vi "FPGA Top - Packet RX Only.vi"() -> ()   [LabVIEW 2017, in "My Network FPGA v1.lvlib"]
uses:
  My Network FPGA v1.lvlib
  <instrlib>/_niInstr/Network/Types/v1/IPv4 Address.ctl
  <instrlib>/_niInstr/Network/Types/v1/MAC Address.ctl
  <instrlib>/_niInstr/Network/Ethernet/MAC/CLIP/v1/Resources.ctl
  <vilib>/Platform/TimedLoop/XDataNode/timing_clust.ctl
  <vilib>/Platform/TimedLoop/XDataNode/nitl_modes.ctl
  <vilib>/Platform/TimedLoop/XDataNode/wakeup.ctl
  <vilib>/rvi/Emulation/niFpgaSctlEmulationGetInTimedLoop.vi
  <vilib>/rvi/Emulation/niFpgaEmulationReportErrorSimple.vi
  <vilib>/rvi/Emulation/niFpgaGetClockAttributes.vi
  <vilib>/rvi/Emulation/niFpgaCriticalErrorInLSC.vi
  <instrlib>/_niInstr/Network/IPv4/UDP/Data Stream/v1/Read Data Stream.vi
  <vilib>/rvi/DataTransferAndStorage/Container/Common/niFpgaContainerExecOnDevCompGetState.vi
  <vilib>/rvi/errors/niFpgaSetErrorForExecOnDevCompSimple.vi
  <vilib>/rvi/eio/common/nirviEmuReportErrorAndStop.vi
  <vilib>/rvi/interface/RandomDataEmulation/nirviRandomDataAcquireLock.vi
  <vilib>/rvi/interface/RandomDataEmulation/nirviRandomDataQueueStore.vi
  <vilib>/rvi/interface/RandomDataEmulation/nirviRandomDataReleaseLock.vi
  <vilib>/rvi/interface/RandomDataEmulation/nirviFPGAContextMergeError.vi
  <vilib>/rvi/interface/RandomDataEmulation/nirviRandomDataCheckExitLoopConditions.vi
  <vilib>/express/rvi/timingcommon/nirviCommon.vi
  <vilib>/rvi/interface/RandomDataEmulation/niFpgaRandomDataHandleErrors.vi
  <vilib>/rvi/eio/common/nirviEmuTemplateMethod_errors.vi
  <vilib>/platform/TimedLoop/XDataNode/XDataNode.xnode
  <vilib>/rvi/DataTransferAndStorage/Container/XNode/niFpgaContainer.xnode
  <vilib>/rvi/FIFO/Fifo_Resource/niFpgaFifoEmulationRefInMultiElement.vi
  <vilib>/eio/EIONode/EIONode.xnode
  <instrlib>/_niInstr/Network/Ethernet/MAC/CLIP/v1/niInstr Ethernet MAC - CLIP v1.lvclass
  <vilib>/Platform/TimedLoop/XDataNode/XDNodeRunTimeDep.lvlib
  <instrlib>/_niInstr/Network/IPv4/UDP/FPGA/v1/niInstr IPv4 UDP FPGA v1.lvlib
  <instrlib>/_niInstr/Network/IPv4/FPGA/v1/niInstr IPv4 FPGA v1.lvlib
  <instrlib>/_niInstr/Network/Ethernet/Utility/v1/FPGA/niInstr Ethernet Utilities FPGA v1.lvlib
  <instrlib>/_niInstr/Network/IPv4/UDP/Data Stream/v1/niInstr IPv4 UDP Data Stream v1.lvclass
  <instrlib>/_niInstr/Network/Ethernet/ARP/v1/FPGA/niInstr Network ARP FPGA v1.lvlib
  <instrlib>/_niInstr/Network/Types/v1/niInstr Network Types v1.lvlib
panel:
  out "aBlockLockPort0":bool
  out "aBlockLockPort1":bool
  out "mgtrefclks_locked":bool
  out "mgtrefclks_valid":bool
  out "posc_complete":bool
  out "sPort0_Power_Good":bool
  out "sPort1_Power_Good":bool
  out "signal_detect_Port0":bool
  out "signal_detect_Port1":bool
  in  "disable IP filtering":bool
  out "byte enables":bool[](array[boolean])
  out "data":u8[](array[numeric])
  in  "Promiscuous?":bool
  in  "MAC local address":T1=[0, 128, 47, 0, 0, 1] format="%.0x"
  in  "IPv4 local address":T2=[0, 0, 0, 0]
  in  "UDP destination port":u16=35311
  # "Network Configuration"
  # "Received Data"
  # "Status"
  # "00802F000001x2^0"
  # "Also see Port 0 RX FIFO"
  # "License Note\nThis example makes use of code under the LGPLv2 license in the Socketed CLIP to support 10 Gigabit Ethernet.  You may find the source and build instructions for this component in the CLIP directory."
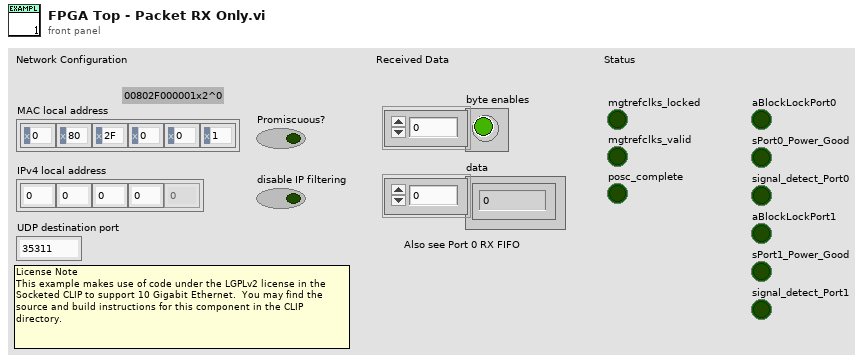
[diagram p1: front panel]
types:
  T1 = typedef "niInstr Network Types v1.lvlib/MAC Address.ctl" = u8[]
  T2 = typedef "niInstr Network Types v1.lvlib/IPv4 Address.ctl" = u8[]
  T3 = typedef "niInstr Ethernet MAC - CLIP v1.lvclass/Resources.ctl" = cluster{"RX":cluster{"TData":refnum<k21>, "TValid":refnum<k21>, "TKeep":refnum<k21>, "TLast":refnum<k21>, "TUser":refnum<k21>}, "TX":cluster{"TData":refnum<k21>, "TValid":refnum<k21>, "TKeep":refnum<k21>, "TLast":refnum<k21>, "TReady":refnum<k21>}, "Pause resources":cluster{"cPauseValuePort":refnum<k21>, "cPauseReqPort":refnum<k21>}, "MAC Clock":refnum<k21>}
  T4 = typedef "XDNodeRunTimeDep.lvlib/timing_clust.ctl" = cluster{"Expected End [f-1]":u64, "Actual End [f-1]":u64, "Finished Late? [f-1]":bool, "Expected End [i-1]":u64, "Actual End [i-1]":u64, "Finished Late? [i-1]":bool, "Expected Start [i]":u64, "Actual Start [i]":u64, "Expected Start [f]":u64, "Actual Start [f]":u64, "Source Name":string, "Structure Name":string, "Period":i64, "Deadline":i64, "Offset":i64, "Start":i64, "Priority":i32, "Timeout":i32, "Mode":T5, "Wakeup Reason":T6, "Error":errorcluster, "Source Type":string, "Secondary Source Type":string, "Global End Time":u64, "Global Start Time":u64, "Frame Duration":u64, "Iteration Duration":u64, "Assigned CPU":i32, "I/O Scan Engine Mode":u32}
  T5 = typedef "XDNodeRunTimeDep.lvlib/nitl_modes.ctl" = enum32{"No Change", "Process missed periods, maintain original phase", "Discard missed periods, maintain original phase", "Process missed periods, ignore original phase", "Discard missed periods, ignore original phase"}
  T6 = typedef "XDNodeRunTimeDep.lvlib/wakeup.ctl" = enum32{"Normal", "Aborted", "Asynchronous wakeup", "Timing source error", "Timed loop error", "Timeout"}
  T7 = typedef "niInstr Ethernet Utilities FPGA v1.lvlib/Network Data Stream.ctl" = cluster{"data":u8[], "data valid":bool, "byte enables":bool[]}
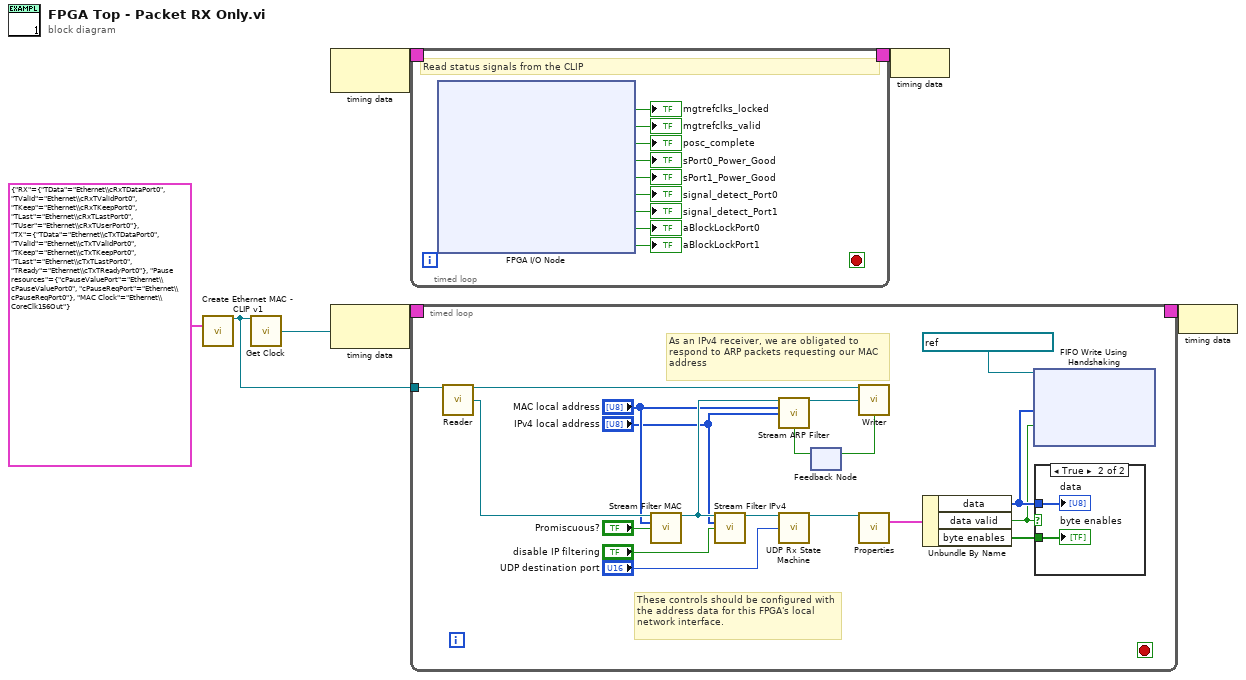
[diagram p0: block diagram]
diagram:
  n1 = call <instrlib>:"Create Ethernet MAC - CLIP v1.vi"("Ethernet AXI4-S Resources"=T3 {"RX"={"TData"="Ethernet\\cRxTDataPort0", "TValid"="Ethernet\\cRxTValidPort0", "TKeep"="Ethernet\\cRxTKeepPort0", "TLast"="Ethernet\\cRxTLastPort0", "TUser"="Ethernet\\cRxTUserPort0"}, "TX"={"TData"="Ethernet\\cTxTDataPort0", "TValid"="Ethernet\\cTxTValidPort0", "TKeep"="Ethernet\\cTxTKeepPort0", "TLast"="Ethernet\\cTxTLastPort0", "TReady"="Ethernet\\cTxTReadyPort0"}, "Pause resources"={"cPauseValuePort"="Ethernet\\cPauseValuePort0", "cPauseReqPort"="Ethernet\\cPauseReqPort0"}, "MAC Clock"="Ethernet\\CoreClk156Out"}) -> ("niInstr Ethernet MAC - CLIP v1.lvclass out"=w4:refnum<class "niInstr Ethernet MAC - CLIP v1.lvclass">)  [unwired: 14 in]
  n2 = call-dynamic "Get Clock.vi"("niInstr Ethernet MAC - CLIP v1.lvclass"=w4) -> ("MAC Clock"=w1:refnum<k21>)  [unwired: 14 in]
  n3 = node-c288() -> (w3:T4)  [unwired: 1 in]
  n4 = node-c288(w1) -> (w7:T4)
  n5 = timed-loop {
    timing: w3 -> [_]
    timing-out: [_] -> w2
    stop <- _ stop-if-true
    # "Read status signals from the CLIP"
    n6 = xnode "FPGA I/O Node"() -> ("Ethernet\\MgtRefClks_Locked"=→"mgtrefclks_locked":bool, "Ethernet\\MgtRefClks_Valid"=→"mgtrefclks_valid":bool, "Ethernet\\POSC_Complete"=→"posc_complete":bool, "Ethernet\\sPort0_Power_Good"=→"sPort0_Power_Good":bool, "Ethernet\\sPort1_Power_Good"=→"sPort1_Power_Good":bool, "Ethernet\\signal_detect_Port0"=→"signal_detect_Port0":bool, "Ethernet\\signal_detect_Port1"=→"signal_detect_Port1":bool, "Ethernet\\aBlockLockPort0"=→"aBlockLockPort0":bool, "Ethernet\\aBlockLockPort1"=→"aBlockLockPort1":bool)  [unwired: 9 in, 9 out]
  }
  n7 = timed-loop {
    timing: w7 -> [_]
    timing-out: [_] -> w6
    tunnel: w4 -> [w35]
    stop <- _ stop-if-true
    # "As an IPv4 receiver, we are obligated to respond to ARP packets requesting our MAC address"
    # "These controls should be configured with the address data for this FPGA's local network interface."
    n8 = call-dynamic "Reader.vi"("niInstr Ethernet MAC - CLIP v1.lvclass 2"=w35) -> ("niInstr Ethernet MAC - CLIP v1.lvclass"=w25:refnum<class "niInstr Ethernet MAC - CLIP v1.lvclass">, "niInstr Ethernet MAC Raw Stream v1.lvclass"=w36:refnum<class "niInstr Ethernet MAC Raw Stream v1.lvclass">)  [unwired: 13 in]
    n9 = call <instrlib>:"Stream Filter MAC.vi"("niInstr Ethernet MAC Raw Stream v1 in"=w36, "MAC Address"="MAC local address", "Promiscuous?"="Promiscuous?") -> ("niInstr Ethernet MAC Data Stream v1 out"=w29:refnum<class "niInstr Ethernet MAC Data Stream v1.lvclass">)  [unwired: 12 in]
    n10 = call <instrlib>:"Stream Filter IPv4.vi"("niInstr Ethernet MAC Data Stream v1 in"=w29, "IP Address"="IPv4 local address", "disable IP filtering"="disable IP filtering") -> ("niInstr IPv4 Data Stream out"=w37:refnum<class "niInstr IPv4 Data Stream v1.lvclass">)  [unwired: 12 in]
    n11 = call <instrlib>:"UDP Rx State Machine.vi"("niInstr IPv4 Data Stream in"=w37, "Dest Port"="UDP destination port") -> ("niInstr IPv4 UDP Data Stream out"=w32:refnum<class "niInstr IPv4 UDP Data Stream v1.lvclass">)  [unwired: 13 in]
    n12 = feedback #1() -> (w26:bool)  [unwired: 1 in]
    n13 = call <instrlib>:"Stream ARP Filter.vi"("niInstr Ethernet MAC Data Stream v1 in"=w29, "MAC Address"="MAC local address", "Local IP"="IPv4 local address", "ready for output"=w26) -> ("niInstr Ethernet MAC Raw Stream v1 out"=w28:refnum<class "niInstr Ethernet MAC Raw Stream v1.lvclass">)  [unwired: 11 in]
    n14 = call-dynamic "Writer.vi"("niInstr Ethernet MAC v1.lvclass"=w25, "niInstr Ethernet MAC Raw Stream v1.lvclass"=w28) -> ("ready for input?"=w27:bool)  [unwired: 12 in, 1 out]
    n15 = feedback-in #1(w27) -> ()
    n16 = call-poly <instrlib>:"Properties.vi"("niInstr IPv4 UDP Data Stream v1.lvclass"=w32) -> ("Data Stream"=w31:T7)  [unwired: 9 in, 1 out]
    n17 = Unbundle By Name(w31) -> ("data"=w20:u8[], "data valid"=w19:bool, "byte enables"=w30:bool[])
    n18 = xnode ("FIFO Write Using Handshaking")("Element"=w20, "Input Valid"=w19, "FIFO In"=refnum<k21> "Port 0 Host RX FIFO") -> ()  [unwired: 2 out]
    n19 = case shown="True" w19 {
      tunnel: w20 -> [_ w39]
      tunnel: w30 -> [_ w38]
      frame False {
      }
      frame True {
        "data" <- w39
        "byte enables" <- w38
      }
    }
  }
  n20 = node-c288(w2) -> ()
  n21 = node-c288(w6) -> ()
